vi "Lab Panel V5.20.vi"() -> ()   [LabVIEW 2013] (continued)
                  tunnel: w4670 -> [w4735 _ _]
                  tunnel: w4669 -> [w4733 _ _]
                  tunnel: w4668 -> [w4724 _ _]
                  tunnel: w4667 -> [w4722 _ _]
                  tunnel: w4666 -> [w4716 _ _]
                  tunnel: w4665 -> [w4714 _ _]
                  tunnel: w4664 -> [_ w4760 _]
                  tunnel: w4663 -> [_ w4758 _]
                  tunnel: w4662 -> [_ w4749 _]
                  tunnel: w4661 -> [_ w4747 _]
                  frame #0 {
                    n2509 = Merge Signals(w4742, w4741) -> (→"LAB01 AMPS":dynamicdata)
                    n2510 = Merge Signals(w4739, w4738) -> (→"LAB01 VOLTS":dynamicdata)
                    n2511 = Merge Signals(w4719, w4718) -> (→"LAB03 VOLTS":dynamicdata)
                    n2512 = Merge Signals(w4736, w4735, w4734, w4733) -> (→"LAB01 deg C":dynamicdata)
                    n2513 = Merge Signals(w4732, w4731) -> (→"LAB02 AMPS":dynamicdata)
                    n2514 = Merge Signals(w4725, w4724, w4723, w4722) -> (→"LAB02 deg C":dynamicdata)
                    n2515 = Merge Signals(w4717, w4716, w4715, w4714) -> (→"LAB03 deg C":dynamicdata)
                    n2516 = Merge Signals(w4729, w4728) -> (→"LAB02 VOLTS":dynamicdata)
                    n2517 = Merge Signals(w4721, w4720) -> (→"LAB03 AMPS":dynamicdata)
                  }
                  frame #1 {
                    n2518 = Merge Signals(w4752, w4751) -> (→"LAB05 VOLTS":dynamicdata)
                    n2519 = Merge Signals(w4765, w4764) -> (→"LAB04 AMPS":dynamicdata)
                    n2520 = Merge Signals(w4754, w4753) -> (→"LAB05 AMPS":dynamicdata)
                    n2521 = Merge Signals(w4750, w4749, w4748, w4747) -> (→"LAB05 deg C":dynamicdata)
                    n2522 = Merge Signals(w4761, w4760, w4759, w4758) -> (→"LAB04 deg C":dynamicdata)
                    n2523 = Merge Signals(w4763, w4762) -> (→"LAB04 VOLTS":dynamicdata)
                  }
                  frame #2 {
                    n2524 = local read "LAB05 VOLTS"() -> (w4773:dynamicdata)
                    n2525 = local read "LAB04 VOLTS"() -> (w4774:dynamicdata)
                    n2526 = local read "LAB02 VOLTS"() -> (w4776:dynamicdata)
                    n2527 = local read "LAB03 VOLTS"() -> (w4775:dynamicdata)
                    n2528 = local read "LAB05 AMPS"() -> (w4779:dynamicdata)
                    n2529 = local read "LAB01 VOLTS"() -> (w4777:dynamicdata)
                    n2530 = local read "LAB04 AMPS"() -> (w4780:dynamicdata)
                    n2531 = local read "LAB03 deg C"() -> (w4769:dynamicdata)
                    n2532 = local read "LAB03 AMPS"() -> (w4781:dynamicdata)
                    n2533 = local read "LAB04 deg C"() -> (w4768:dynamicdata)
                    n2534 = local read "LAB05 deg C"() -> (w4767:dynamicdata)
                    n2535 = local read "LAB02 AMPS"() -> (w4782:dynamicdata)
                    n2536 = local read "LAB02 deg C"() -> (w4770:dynamicdata)
                    n2537 = local read "LAB01 deg C"() -> (w4771:dynamicdata)
                    n2538 = local read "LAB01 AMPS"() -> (w4783:dynamicdata)
                    n2539 = Merge Signals(w4771, w4770, w4769, w4768, w4767) -> (w4766:dynamicdata)
                    n2540 = Merge Signals(w4783, w4782, w4781, w4780, w4779) -> (w4778:dynamicdata)
                    n2541 = Merge Signals(w4777, w4776, w4775, w4774, w4773) -> (w4772:dynamicdata)
                    n2542 = global write "Global display 3.vi" "graph volts"(w4772) -> ()
                    n2543 = global write "Global display 3.vi" "graph deg C"(w4766) -> ()
                    n2544 = global write "Global display 3.vi" "graph amps"(w4778) -> ()
                  }
                }
              }
            }
          }
          frame #14 {
            # "check for amps fail"
            # "check for cycle test & temperature rise fail conditions"
            n2545 = local read "jig cycle"() -> (w4807:dbl)
            n2546 = local read "on loops"() -> (w4810:dbl)
            n2547 = local read "jig cycle"() -> (w4812:dbl)
            n2548 = Add(x=w4810, y=3.0) -> (x+y=w4808:dbl)
            n2549 = Equal?(x=w4807, y=w4808) -> (x = y?=w4803:bool)
            n2550 = local read "Fail Loops"() -> (w4784:dbl)
            n2551 = Equal?(x=w4812, y=1.0) -> (x = y?=w4805:bool)
            n2552 = global write "Global 1.vi" "fail count"(w4784) -> ()
            n2553 = stacked-sequence {
              tunnel: w4806 -> [w4815 _ _ _ _ _ _ _ _ _]
              tunnel: w4805 -> [w4816 w4836 w4856 w4876 w4896 w4916 w4936 w4956 w4976 w4996]
              tunnel: w4804 -> [w4813 _ _ _ _ _ _ _ _ _]
              tunnel: w4803 -> [w4814 w4835 w4855 w4875 w4895 w4915 w4935 w4955 w4975 w4995]
              tunnel: w4802 -> [_ w4834 _ _ _ _ _ _ _ _]
              tunnel: w4801 -> [_ w4833 _ _ _ _ _ _ _ _]
              tunnel: w4800 -> [_ _ w4854 _ _ _ _ _ _ _]
              tunnel: w4799 -> [_ _ w4853 _ _ _ _ _ _ _]
              tunnel: w4798 -> [_ _ _ w4874 _ _ _ _ _ _]
              tunnel: w4797 -> [_ _ _ w4873 _ _ _ _ _ _]
              tunnel: w4796 -> [_ _ _ _ w4894 _ _ _ _ _]
              tunnel: w4795 -> [_ _ _ _ w4893 _ _ _ _ _]
              tunnel: w4794 -> [_ _ _ _ _ w4914 _ _ _ _]
              tunnel: w4793 -> [_ _ _ _ _ w4913 _ _ _ _]
              tunnel: w4792 -> [_ _ _ _ _ _ w4934 _ _ _]
              tunnel: w4791 -> [_ _ _ _ _ _ w4933 _ _ _]
              tunnel: w4790 -> [_ _ _ _ _ _ _ w4954 _ _]
              tunnel: w4789 -> [_ _ _ _ _ _ _ w4953 _ _]
              tunnel: w4788 -> [_ _ _ _ _ _ _ _ w4974 _]
              tunnel: w4787 -> [_ _ _ _ _ _ _ _ w4973 _]
              tunnel: w4786 -> [_ _ _ _ _ _ _ _ _ w4994]
              tunnel: w4785 -> [_ _ _ _ _ _ _ _ _ w4993]
              frame #0 {
                # "LAB01-1"
                n2554 = case shown="True" w4813 {
                  tunnel: w4816 -> [_ w4829]
                  tunnel: w4815 -> [_ w4826]
                  tunnel: w4814 -> [_ w4825]
                  frame False {
                  }
                  frame True {
                    n2555 = local read "TEMP START LAB01-1"() -> (w4831:cluster{"TL":dbl, "TN":dbl})
                    n2556 = local read "RESULT LAB01-1"() -> (w4820:bool)
                    n2557 = local read "FAIL LAB01-1"() -> (w4823:cluster{"LO":dbl, "HI":dbl})
                    n2558 = local read "SET LAB01-1"() -> (w4827:T5)
                    n2559 = local read "TDMS LAB01-1"() -> (w4830:refnum<k34>)
                    n2560 = local read "DISP LAB01-1"() -> (w4828:T4)
                    n2561 = local read "SIG LAB01-1"() -> (w4832:T2)
                    n2562 = Bundle("FAIL LAB01-1"=w4823, "SIG LAB01-1"=w4832, "TEMP START LAB01-1"=w4831, "DISP LAB01-1"=w4828, "SET LAB01-1"=w4827, "TDMS LAB01-1"=w4830) -> (w4817:T32)  [unwired: 1 in]
                    n2563 = call "sub vi - cycle&temp fail v7.vi"("Amps Lo?"=w4829, "Input Cluster"=w4817, "SELECT"=w4826, "Amps Hi?"=w4825, "Result In"=w4820) -> ("(FAIL) out"=w4822:cluster{"FAIL LO":dbl, "FAIL HI":dbl}, "(DISP) out"=w4818:T4, "T-RISE"=w4819:cluster{"T-RISE (L)":dbl, "T-RISE (N)":dbl}, "Result Out"=w4821:bool, "file error"=w4824:errorcluster)  [unwired: 10 in]
                    n2564 = local write "TEMP RISE LAB01-1"(w4819) -> ()
                    n2565 = local write "FAIL LAB01-1"(w4822) -> ()
                    n2566 = local write "DISP LAB01-1"(w4818) -> ()
                    n2567 = local write "RESULT LAB01-1"(w4821) -> ()
                    n2568 = local write "data file error"(w4824) -> ()
                  }
                }
              }
              frame #1 {
                # "LAB01-2"
                n2569 = case shown="True" w4834 {
                  tunnel: w4836 -> [_ w4849]
                  tunnel: w4833 -> [_ w4846]
                  tunnel: w4835 -> [_ w4845]
                  frame False {
                  }
                  frame True {
                    n2570 = local read "TEMP START LAB01-2"() -> (w4851:cluster{"TL":dbl, "TN":dbl})
                    n2571 = local read "FAIL LAB01-2"() -> (w4842:cluster{"LO":dbl, "HI":dbl})
                    n2572 = local read "SET LAB01-2"() -> (w4847:T5)
                    n2573 = local read "TDMS LAB01-2"() -> (w4850:refnum<k34>)
                    n2574 = local read "DISP LAB01-2"() -> (w4848:T4)
                    n2575 = local read "RESULT LAB01-2"() -> (w4839:bool)
                    n2576 = local read "SIG LAB01-2"() -> (w4852:T2)
                    n2577 = Bundle("FAIL LAB01-2"=w4842, "SIG LAB01-2"=w4852, "TEMP START LAB01-2"=w4851, "DISP LAB01-2"=w4848, "SET LAB01-2"=w4847, "TDMS LAB01-2"=w4850) -> (w4837:T33)  [unwired: 1 in]
                    n2578 = call "sub vi - cycle&temp fail v7.vi"("Amps Lo?"=w4849, "Input Cluster"=w4837, "SELECT"=w4846, "Amps Hi?"=w4845, "Result In"=w4839) -> ("(FAIL) out"=w4841:cluster{"FAIL LO":dbl, "FAIL HI":dbl}, "(DISP) out"=w4844:T4, "T-RISE"=w4838:cluster{"T-RISE (L)":dbl, "T-RISE (N)":dbl}, "Result Out"=w4840:bool, "file error"=w4843:errorcluster)  [unwired: 10 in]
                    n2579 = local write "TEMP RISE LAB01-2"(w4838) -> ()
                    n2580 = local write "FAIL LAB01-2"(w4841) -> ()
                    n2581 = local write "DISP LAB01-2"(w4844) -> ()
                    n2582 = local write "RESULT LAB01-2"(w4840) -> ()
                    n2583 = local write "data file error"(w4843) -> ()
                  }
                }
              }
              frame #2 {
                # "LAB02-1"
                n2584 = case shown="True" w4854 {
                  tunnel: w4856 -> [_ w4869]
                  tunnel: w4853 -> [_ w4866]
                  tunnel: w4855 -> [_ w4865]
                  frame False {
                  }
                  frame True {
                    n2585 = local read "TEMP START LAB02-1"() -> (w4871:cluster{"TL":dbl, "TN":dbl})
                    n2586 = local read "FAIL LAB02-1"() -> (w4862:cluster{"LO":dbl, "HI":dbl})
                    n2587 = local read "SET LAB02-1"() -> (w4867:T5)
                    n2588 = local read "TDMS LAB02-1"() -> (w4870:refnum<k34>)
                    n2589 = local read "DISP LAB02-1"() -> (w4868:T4)
                    n2590 = local read "SIG LAB02-1"() -> (w4872:T2)
                    n2591 = local read "RESULT LAB02-1"() -> (w4859:bool)
                    n2592 = Bundle("FAIL LAB02-1"=w4862, "SIG LAB02-1"=w4872, "TEMP START LAB02-1"=w4871, "DISP LAB02-1"=w4868, "SET LAB02-1"=w4867, "TDMS LAB02-1"=w4870) -> (w4857:T34)  [unwired: 1 in]
                    n2593 = call "sub vi - cycle&temp fail v7.vi"("Amps Lo?"=w4869, "Input Cluster"=w4857, "SELECT"=w4866, "Amps Hi?"=w4865, "Result In"=w4859) -> ("(FAIL) out"=w4861:cluster{"FAIL LO":dbl, "FAIL HI":dbl}, "(DISP) out"=w4864:T4, "T-RISE"=w4858:cluster{"T-RISE (L)":dbl, "T-RISE (N)":dbl}, "Result Out"=w4860:bool, "file error"=w4863:errorcluster)  [unwired: 10 in]
                    n2594 = local write "TEMP RISE LAB02-1"(w4858) -> ()
                    n2595 = local write "FAIL LAB02-1"(w4861) -> ()
                    n2596 = local write "DISP LAB02-1"(w4864) -> ()
                    n2597 = local write "RESULT LAB02-1"(w4860) -> ()
                    n2598 = local write "data file error"(w4863) -> ()
                  }
                }
              }
              frame #3 {
                # "LAB02-2"
                n2599 = case shown="True" w4874 {
                  tunnel: w4876 -> [_ w4889]
                  tunnel: w4873 -> [_ w4886]
                  tunnel: w4875 -> [_ w4885]
                  frame False {
                  }
                  frame True {
                    n2600 = local read "TEMP START LAB02-2"() -> (w4891:cluster{"TL":dbl, "TN":dbl})
                    n2601 = local read "FAIL LAB02-2"() -> (w4882:cluster{"LO":dbl, "HI":dbl})
                    n2602 = local read "SET LAB02-2"() -> (w4887:T5)
                    n2603 = local read "TDMS LAB02-2"() -> (w4890:refnum<k34>)
                    n2604 = local read "DISP LAB02-2"() -> (w4888:T4)
                    n2605 = local read "SIG LAB02-2"() -> (w4892:T2)
                    n2606 = local read "RESULT LAB02-2"() -> (w4879:bool)
                    n2607 = Bundle("FAIL LAB02-2"=w4882, "SIG LAB02-2"=w4892, "TEMP START LAB02-2"=w4891, "DISP LAB02-2"=w4888, "SET LAB02-2"=w4887, "TDMS LAB02-2"=w4890) -> (w4877:T35)  [unwired: 1 in]
                    n2608 = call "sub vi - cycle&temp fail v7.vi"("Amps Lo?"=w4889, "Input Cluster"=w4877, "SELECT"=w4886, "Amps Hi?"=w4885, "Result In"=w4879) -> ("(FAIL) out"=w4881:cluster{"FAIL LO":dbl, "FAIL HI":dbl}, "(DISP) out"=w4884:T4, "T-RISE"=w4878:cluster{"T-RISE (L)":dbl, "T-RISE (N)":dbl}, "Result Out"=w4880:bool, "file error"=w4883:errorcluster)  [unwired: 10 in]
                    n2609 = local write "TEMP RISE LAB02-2"(w4878) -> ()
                    n2610 = local write "FAIL LAB02-2"(w4881) -> ()
                    n2611 = local write "DISP LAB02-2"(w4884) -> ()
                    n2612 = local write "RESULT LAB02-2"(w4880) -> ()
                    n2613 = local write "data file error"(w4883) -> ()
                  }
                }
              }
              frame #4 {
                # "LAB03-1"
                n2614 = case shown="True" w4894 {
                  tunnel: w4896 -> [_ w4909]
                  tunnel: w4893 -> [_ w4906]
                  tunnel: w4895 -> [_ w4905]
                  frame False {
                  }
                  frame True {
                    n2615 = local read "TEMP START LAB03-1"() -> (w4911:cluster{"TL":dbl, "TN":dbl})
                    n2616 = local read "FAIL LAB03-1"() -> (w4902:cluster{"LO":dbl, "HI":dbl})
                    n2617 = local read "SET LAB03-1"() -> (w4907:T5)
                    n2618 = local read "TDMS LAB03-1"() -> (w4910:refnum<k34>)
                    n2619 = local read "DISP LAB03-1"() -> (w4908:T4)
                    n2620 = local read "SIG LAB03-1"() -> (w4912:T2)
                    n2621 = local read "RESULT LAB03-1"() -> (w4899:bool)
                    n2622 = Bundle("FAIL LAB03-1"=w4902, "SIG LAB03-1"=w4912, "TEMP START LAB03-1"=w4911, "DISP LAB03-1"=w4908, "SET LAB03-1"=w4907, "TDMS LAB03-1"=w4910) -> (w4897:T36)  [unwired: 1 in]
                    n2623 = call "sub vi - cycle&temp fail v7.vi"("Amps Lo?"=w4909, "Input Cluster"=w4897, "SELECT"=w4906, "Amps Hi?"=w4905, "Result In"=w4899) -> ("(FAIL) out"=w4901:cluster{"FAIL LO":dbl, "FAIL HI":dbl}, "(DISP) out"=w4904:T4, "T-RISE"=w4898:cluster{"T-RISE (L)":dbl, "T-RISE (N)":dbl}, "Result Out"=w4900:bool, "file error"=w4903:errorcluster)  [unwired: 10 in]
                    n2624 = local write "TEMP RISE LAB03-1"(w4898) -> ()
                    n2625 = local write "FAIL LAB03-1"(w4901) -> ()
                    n2626 = local write "DISP LAB03-1"(w4904) -> ()
                    n2627 = local write "RESULT LAB03-1"(w4900) -> ()
                    n2628 = local write "data file error"(w4903) -> ()
                  }
                }
              }
              frame #5 {
                # "LAB03-2"
                n2629 = case shown="True" w4914 {
                  tunnel: w4916 -> [_ w4929]
                  tunnel: w4913 -> [_ w4926]
                  tunnel: w4915 -> [_ w4925]
                  frame False {
                  }
                  frame True {
                    n2630 = local read "TEMP START LAB03-2"() -> (w4931:cluster{"TL":dbl, "TN":dbl})
                    n2631 = local read "FAIL LAB03-2"() -> (w4922:cluster{"LO":dbl, "HI":dbl})
                    n2632 = local read "SET LAB03-2"() -> (w4927:T5)
                    n2633 = local read "TDMS LAB03-2"() -> (w4930:refnum<k34>)
                    n2634 = local read "DISP LAB03-2"() -> (w4928:T4)
                    n2635 = local read "RESULT LAB03-2"() -> (w4919:bool)
                    n2636 = local read "SIG LAB03-2"() -> (w4932:T2)
                    n2637 = Bundle("FAIL LAB03-2"=w4922, "SIG LAB03-2"=w4932, "TEMP START LAB03-2"=w4931, "DISP LAB03-2"=w4928, "SET LAB03-2"=w4927, "TDMS LAB03-2"=w4930) -> (w4917:T37)  [unwired: 1 in]
                    n2638 = call "sub vi - cycle&temp fail v7.vi"("Amps Lo?"=w4929, "Input Cluster"=w4917, "SELECT"=w4926, "Amps Hi?"=w4925, "Result In"=w4919) -> ("(FAIL) out"=w4921:cluster{"FAIL LO":dbl, "FAIL HI":dbl}, "(DISP) out"=w4924:T4, "T-RISE"=w4918:cluster{"T-RISE (L)":dbl, "T-RISE (N)":dbl}, "Result Out"=w4920:bool, "file error"=w4923:errorcluster)  [unwired: 10 in]
                    n2639 = local write "FAIL LAB03-2"(w4921) -> ()
                    n2640 = local write "TEMP RISE LAB03-2"(w4918) -> ()
                    n2641 = local write "DISP LAB03-2"(w4924) -> ()
                    n2642 = local write "RESULT LAB03-2"(w4920) -> ()
                    n2643 = local write "data file error"(w4923) -> ()
                  }
                }
              }
              frame #6 {
                # "LAB04-1"
                n2644 = case shown="True" w4934 {
                  tunnel: w4936 -> [_ w4949]
                  tunnel: w4933 -> [_ w4946]
                  tunnel: w4935 -> [_ w4945]
                  frame False {
                  }
                  frame True {
                    n2645 = local read "TEMP START LAB04-1"() -> (w4951:cluster{"TL":dbl, "TN":dbl})
                    n2646 = local read "FAIL LAB04-1"() -> (w4942:cluster{"LO":dbl, "HI":dbl})
                    n2647 = local read "SET LAB04-1"() -> (w4947:T5)
                    n2648 = local read "TDMS LAB04-1"() -> (w4950:refnum<k34>)
                    n2649 = local read "DISP LAB04-1"() -> (w4948:T4)
                    n2650 = local read "SIG LAB04-1"() -> (w4952:T2)
                    n2651 = local read "RESULT LAB04-1"() -> (w4939:bool)
                    n2652 = Bundle("FAIL LAB04-1"=w4942, "SIG LAB04-1"=w4952, "TEMP START LAB04-1"=w4951, "DISP LAB04-1"=w4948, "SET LAB04-1"=w4947, "TDMS LAB04-1"=w4950) -> (w4937:T38)  [unwired: 1 in]
                    n2653 = call "sub vi - cycle&temp fail v7.vi"("Amps Lo?"=w4949, "Input Cluster"=w4937, "SELECT"=w4946, "Amps Hi?"=w4945, "Result In"=w4939) -> ("(FAIL) out"=w4941:cluster{"FAIL LO":dbl, "FAIL HI":dbl}, "(DISP) out"=w4944:T4, "T-RISE"=w4938:cluster{"T-RISE (L)":dbl, "T-RISE (N)":dbl}, "Result Out"=w4940:bool, "file error"=w4943:errorcluster)  [unwired: 10 in]
                    n2654 = local write "FAIL LAB04-1"(w4941) -> ()
                    n2655 = local write "TEMP RISE LAB04-1"(w4938) -> ()
                    n2656 = local write "DISP LAB04-1"(w4944) -> ()
                    n2657 = local write "RESULT LAB04-1"(w4940) -> ()
                    n2658 = local write "data file error"(w4943) -> ()
                  }
                }
              }
              frame #7 {
                # "LAB04-2"
                n2659 = case shown="True" w4954 {
                  tunnel: w4956 -> [_ w4969]
                  tunnel: w4953 -> [_ w4966]
                  tunnel: w4955 -> [_ w4965]
                  frame False {
                  }
                  frame True {
                    n2660 = local read "TEMP START LAB04-2"() -> (w4971:cluster{"TL":dbl, "TN":dbl})
                    n2661 = local read "FAIL LAB04-2"() -> (w4962:cluster{"LO":dbl, "HI":dbl})
                    n2662 = local read "SET LAB04-2"() -> (w4967:T5)
                    n2663 = local read "TDMS LAB04-2"() -> (w4970:refnum<k34>)
                    n2664 = local read "DISP LAB04-2"() -> (w4968:T4)
                    n2665 = local read "SIG LAB04-2"() -> (w4972:T2)
                    n2666 = local read "RESULT LAB04-2"() -> (w4959:bool)
                    n2667 = Bundle("FAIL LAB04-2"=w4962, "SIG LAB04-2"=w4972, "TEMP START LAB04-2"=w4971, "DISP LAB04-2"=w4968, "SET LAB04-2"=w4967, "TDMS LAB04-2"=w4970) -> (w4957:T39)  [unwired: 1 in]
                    n2668 = call "sub vi - cycle&temp fail v7.vi"("Amps Lo?"=w4969, "Input Cluster"=w4957, "SELECT"=w4966, "Amps Hi?"=w4965, "Result In"=w4959) -> ("(FAIL) out"=w4961:cluster{"FAIL LO":dbl, "FAIL HI":dbl}, "(DISP) out"=w4964:T4, "T-RISE"=w4958:cluster{"T-RISE (L)":dbl, "T-RISE (N)":dbl}, "Result Out"=w4960:bool, "file error"=w4963:errorcluster)  [unwired: 10 in]
                    n2669 = local write "TEMP RISE LAB04-2"(w4958) -> ()
                    n2670 = local write "FAIL LAB04-2"(w4961) -> ()
                    n2671 = local write "DISP LAB04-2"(w4964) -> ()
                    n2672 = local write "RESULT LAB04-2"(w4960) -> ()
                    n2673 = local write "data file error"(w4963) -> ()
                  }
                }
              }
              frame #8 {
                # "LAB05-1"
                n2674 = case shown="True" w4974 {
                  tunnel: w4976 -> [_ w4989]
                  tunnel: w4973 -> [_ w4986]
                  tunnel: w4975 -> [_ w4985]
                  frame False {
                  }
                  frame True {
                    n2675 = local read "TEMP START LAB05-1"() -> (w4991:cluster{"TL":dbl, "TN":dbl})
                    n2676 = local read "FAIL LAB05-1"() -> (w4982:cluster{"LO":dbl, "HI":dbl})
                    n2677 = local read "SET LAB05-1"() -> (w4987:T5)
                    n2678 = local read "TDMS LAB05-1"() -> (w4990:refnum<k34>)
                    n2679 = local read "DISP LAB05-1"() -> (w4988:T4)
                    n2680 = local read "SIG LAB05-1"() -> (w4992:T2)
                    n2681 = local read "RESULT LAB05-1"() -> (w4979:bool)
                    n2682 = Bundle("FAIL LAB05-1"=w4982, "SIG LAB05-1"=w4992, "TEMP START LAB05-1"=w4991, "DISP LAB05-1"=w4988, "SET LAB05-1"=w4987, "TDMS LAB05-1"=w4990) -> (w4977:T40)  [unwired: 1 in]
                    n2683 = call "sub vi - cycle&temp fail v7.vi"("Amps Lo?"=w4989, "Input Cluster"=w4977, "SELECT"=w4986, "Amps Hi?"=w4985, "Result In"=w4979) -> ("(FAIL) out"=w4981:cluster{"FAIL LO":dbl, "FAIL HI":dbl}, "(DISP) out"=w4984:T4, "T-RISE"=w4978:cluster{"T-RISE (L)":dbl, "T-RISE (N)":dbl}, "Result Out"=w4980:bool, "file error"=w4983:errorcluster)  [unwired: 10 in]
                    n2684 = local write "TEMP RISE LAB05-1"(w4978) -> ()
                    n2685 = local write "FAIL LAB05-1"(w4981) -> ()
                    n2686 = local write "DISP LAB05-1"(w4984) -> ()
                    n2687 = local write "RESULT LAB05-1"(w4980) -> ()
                    n2688 = local write "data file error"(w4983) -> ()
                  }
                }
              }
              frame #9 {
                # "LAB05-2"
                n2689 = case shown="True" w4994 {
                  tunnel: w4996 -> [_ w5009]
                  tunnel: w4993 -> [_ w5006]
                  tunnel: w4995 -> [_ w5005]
                  frame False {
                  }
                  frame True {
                    n2690 = local read "TEMP START LAB05-2"() -> (w5011:cluster{"TL":dbl, "TN":dbl})
                    n2691 = local read "FAIL LAB05-2"() -> (w5002:cluster{"LO":dbl, "HI":dbl})
                    n2692 = local read "SET LAB05-2"() -> (w5007:T5)
                    n2693 = local read "TDMS LAB05-2"() -> (w5010:refnum<k34>)
                    n2694 = local read "DISP LAB05-2"() -> (w5008:T4)
                    n2695 = local read "SIG LAB05-2"() -> (w5012:T2)
                    n2696 = local read "RESULT LAB05-2"() -> (w4999:bool)
                    n2697 = Bundle("FAIL LAB05-2"=w5002, "SIG LAB05-2"=w5012, "TEMP START LAB05-2"=w5011, "DISP LAB05-2"=w5008, "SET LAB05-2"=w5007, "TDMS LAB05-2"=w5010) -> (w4997:T41)  [unwired: 1 in]
                    n2698 = call "sub vi - cycle&temp fail v7.vi"("Amps Lo?"=w5009, "Input Cluster"=w4997, "SELECT"=w5006, "Amps Hi?"=w5005, "Result In"=w4999) -> ("(FAIL) out"=w5001:cluster{"FAIL LO":dbl, "FAIL HI":dbl}, "(DISP) out"=w5004:T4, "T-RISE"=w4998:cluster{"T-RISE (L)":dbl, "T-RISE (N)":dbl}, "Result Out"=w5000:bool, "file error"=w5003:errorcluster)  [unwired: 10 in]
                    n2699 = local write "TEMP RISE LAB05-2"(w4998) -> ()
                    n2700 = local write "FAIL LAB05-2"(w5001) -> ()
                    n2701 = local write "DISP LAB05-2"(w5004) -> ()
                    n2702 = local write "RESULT LAB05-2"(w5000) -> ()
                    n2703 = local write "data file error"(w5003) -> ()
                  }
                }
              }
            }
          }
          frame #15 {
            # "run calibration routine"
            n2704 = local read "SET (cal)"() -> (w5013:bool)
            n2705 = case shown="True" w5013 {
              frame False {
              }
              frame True {
                n2706 = stacked-sequence {
                  seq-local: [w5014 _ _] -> [_ w5016 _]
                  frame #0 {
                    n2707 = call "CALIBRATION PASSWORD"() -> ("PASSWORD"=w5014:string)  [unwired: 17 in, 2 out]
                  }
                  frame #1 {
                    n2708 = Equal?(x=w5016, y="7777") -> (x = y?=w5015:bool)
                    n2709 = case shown="True" w5015 {
                      frame False {
                      }
                      frame True {
                        n2710 = stacked-sequence {
                          frame #0 {
                            n2711 = local read "Temp Test Cal"() -> (w5018:dbl)
                            n2712 = call "sub vi - calibration v1.vi"("Temp Test Cal"=w5018) -> ()  [unwired: 11 in]
                          }
                          frame #1 {
                            n2713 = call "sub vi - get calibration values v1.vi"() -> ("TEMP REF CAL"=w5019:dbl, "LAB01 (CAL)"=w5024:T14, "LAB02 (CAL)"=w5023:T15, "LAB03 (CAL)"=w5022:T14, "LAB04 (CAL)"=w5021:T14, "calibration file error out"=w5025:errorcluster, "LAB05 (CAL)"=w5020:T14)  [unwired: 9 in]
                            n2714 = local write "TEMP REF cal"(w5019) -> ()
                            n2715 = local write "cal file error out"(w5025) -> ()
                            n2716 = local write "CAL LAB04"(w5021) -> ()
                            n2717 = local write "CAL LAB05"(w5020) -> ()
                            n2718 = local write "CAL LAB01"(w5024) -> ()
                            n2719 = local write "CAL LAB02"(w5023) -> ()
                            n2720 = local write "CAL LAB03"(w5022) -> ()
                          }
                        }
                      }
                    }
                  }
                  frame #2 {
                    n2721 = local write "SET (cal)"(FALSE) -> ()
                  }
                }
              }
            }
          }
          frame #16 {
            # "save certain settings to file"
            n2722 = String To Path(string="c:\\crabtree\\Set Up\\") -> (path=w5028:path)
            n2723 = Build Path(base path=w5028, name or relative path="settings.bin") -> (appended path=w5030:path)
            n2724 = Build Path(base path=w5028, name or relative path="mail.bin") -> (appended path=w5027:path)
            n2725 = Create Folder(path (use dialog)=w5028) -> (error out=w5033:errorcluster)  [unwired: 2 in, 2 out]
            n2726 = call <vilib>:"Clear Errors.vi"("error in (no error)"=w5033) -> ()  [unwired: 6 in, 1 out]
            n2727 = stacked-sequence {
              seq-local: [w5045 _] -> [_ w5058]
              tunnel: w5030 -> [_ w5059]
              tunnel: w5027 -> [_ w5057]
              frame #0 {
                n2728 = local read "C drive data root dir"() -> (w5044:path)
                n2729 = local read "Select COM port"() -> (w5041:refnum<visa-resource-name>)
                n2730 = local read "Network Directory"() -> (w5050:path)
                n2731 = local read "SET LAB05-2"() -> (w5049:T5)
                n2732 = local read "SET LAB05-1"() -> (w5048:T5)
                n2733 = local read "SET LAB04-2"() -> (w5047:T5)
                n2734 = local read "SET LAB03-2"() -> (w5051:T5)
                n2735 = local read "SET LAB04-1"() -> (w5046:T5)
                n2736 = local read "SET LAB03-1"() -> (w5052:T5)
                n2737 = local read "SET LAB02-2"() -> (w5053:T5)
                n2738 = local read "SET LAB02-1"() -> (w5054:T5)
                n2739 = local read "SET LAB01-2"() -> (w5055:T5)
                n2740 = local read "Temp Delay Lps"() -> (w5040:dbl)
                n2741 = local read "Amps Fail level"() -> (w5036:dbl)
                n2742 = local read "Temp Test Cal"() -> (w5037:dbl)
                n2743 = local read "SET LAB01-1"() -> (w5056:T5)
                n2744 = local read "Mail Test File To:"() -> (w5035:string)
                n2745 = local read "Temp Value"() -> (w5039:dbl)
                n2746 = local read "Fail Loops"() -> (w5038:dbl)
                n2747 = local read "Mail Test Fail"() -> (w5034:bool)
                n2748 = local read "RATE (Hz)"() -> (w5043:dbl)
                n2749 = local read "SAMPLES"() -> (w5042:dbl)
                n2750 = Bundle("SET LAB01-1"=w5056, "SET LAB01-2"=w5055, "SET LAB02-1"=w5054, "SET LAB02-2"=w5053, "SET LAB03-1"=w5052, "SET LAB03-2"=w5051, "SET LAB04-1"=w5046, "SET LAB04-2"=w5047, "SET LAB05-1"=w5048, "SET LAB05-2"=w5049, "Network Directory"=w5050, "C drive data root dir"=w5044, "RATE (Hz)"=w5043, "SAMPLES"=w5042, "Select COM port"=w5041, "Temp Delay Lps"=w5040, "Temp Value"=w5039, "Fail Loops"=w5038, "Temp Test Cal"=w5037, "Amps Fail level"=w5036, "Mail Test File To:"=w5035, "Mail Test Fail"=w5034) -> (w5045:T22)  [unwired: 1 in]
              }
              frame #1 {
                n2751 = event shown="[1] \"SET LAB01-1\", \"SET LAB01-2\", \"SET LAB02-1\", \"SET LAB02-2\", \"SET LAB03-1\", \"SET LAB03-2\", \"SET LAB04-1\", \"SET LAB04-2\", \"SET LAB05-1\", \"SET LAB05-2\", \"Network Directory\", \"C drive data root dir\", \"RATE (Hz)\", \"SAMPLES\", \"Select COM port\", \"Temp Delay Lps\", \"Temp Value\", \"Fail Loops\", \"Temp Test Cal\", \"Amps Fail level\", \"Mail Test File To:\", \"Mail Test Fail\": Value Change" {
                  selector: _ -> [_ _ _]
                  dyn-events: _ -> [_ _ _]
                  timeout: 10.0 -> [_ _ _]
                  tunnel: w5059 -> [_ w5061 _]
                  tunnel: w5058 -> [_ w5062 _]
                  tunnel: w5057 -> [_ _ w5073]
                  event Timeout {
                    n2752 = event-data() -> ()  [unwired: 1 in, 3 out]
                  }
                  event "SET LAB01-1", "SET LAB01-2", "SET LAB02-1", "SET LAB02-2", "SET LAB03-1", "SET LAB03-2", "SET LAB04-1", "SET LAB04-2", "SET LAB05-1", "SET LAB05-2", "Network Directory", "C drive data root dir", "RATE (Hz)", "SAMPLES", "Select COM port", "Temp Delay Lps", "Temp Value", "Fail Loops", "Temp Test Cal", "Amps Fail level", "Mail Test File To:", "Mail Test Fail": Value Change {
                    n2753 = event-data() -> ()  [unwired: 1 in, 6 out]
                    n2754 = Open/Create/Replace File(file path (use dialog)=w5061, operation (0:open)=T21."replace or create") -> (refnum out=w5067:refnum<file>, error out=w5066:errorcluster)  [unwired: 4 in, 1 out]
                    n2755 = Write to Binary File(file (use dialog)=w5067, data=w5062, error in=w5066) -> (refnum out=w5065:refnum<file>, error out=w5064:errorcluster)  [unwired: 3 in, 1 out]
                    n2756 = Close File(refnum=w5065, error in=w5064) -> (error out=w5063:errorcluster)  [unwired: 1 out]
                    n2757 = local write "data file error"(w5063) -> ()
                  }
                  event "MAIL SETTINGS.OUT SERVER ADDRESS", "MAIL SETTINGS.FROM ACCOUNT", "MAIL SETTINGS.USER NAME", "MAIL SETTINGS.PASSWORD", "Auto Mail Send", "TO (string):": Value Change {
                    n2758 = event-data() -> ()  [unwired: 1 in, 6 out]
                    n2759 = local read "MAIL SETTINGS"() -> (w5072:T7)
                    n2760 = local read "Auto Mail Send"() -> (w5070:bool)
                    n2761 = local read "TO (string):"() -> (w5069:string)
                    n2762 = Open/Create/Replace File(file path (use dialog)=w5073, operation (0:open)=T21."replace or create") -> (refnum out=w5078:refnum<file>, error out=w5077:errorcluster)  [unwired: 4 in, 1 out]
                    n2763 = Bundle("MAIL SETTINGS"=w5072, "Auto Mail Send"=w5070, "TO (string):"=w5069) -> (w5071:T42)  [unwired: 1 in]
                    n2764 = Write to Binary File(file (use dialog)=w5078, data=w5071, error in=w5077) -> (refnum out=w5076:refnum<file>, error out=w5075:errorcluster)  [unwired: 3 in, 1 out]
                    n2765 = Close File(refnum=w5076, error in=w5075) -> (error out=w5074:errorcluster)  [unwired: 1 out]
                    n2766 = local write "data file error"(w5074) -> ()
                  }
                }
              }
            }
          }
          frame #17 {
            # "mail control"
            n2767 = local read "MAIL SETTINGS"() -> (w5095:T7)
            n2768 = local read "Auto Mail Send"() -> (w5081:bool)
            n2769 = Unbundle(w5095) -> ("OUT SERVER ADDRESS"=w5094:string, "FROM ACCOUNT"=w5093:string, "TEST MAIL"=w5092:bool)  [unwired: 4 out]
            n2770 = stacked-sequence {
              tunnel: "TO (string):" -> [_ w5134]
              tunnel: w5095 -> [w5100 w5133]
              tunnel: w5094 -> [w5099 w5132]
              tunnel: w5093 -> [w5098 w5131]
              tunnel: w5092 -> [w5097 _]
              tunnel: w5081 -> [_ w5130]
              tunnel: w5091 -> [_ w5129]
              tunnel: w5090 -> [_ w5128]
              tunnel: w5089 -> [_ w5127]
              tunnel: w5088 -> [_ w5126]
              tunnel: w5087 -> [_ w5125]
              tunnel: w5086 -> [_ w5124]
              tunnel: w5085 -> [_ w5123]
              tunnel: w5084 -> [_ w5122]
              tunnel: w5083 -> [_ w5121]
              tunnel: w5082 -> [_ w5120]
              tunnel: "TO (string):" -> [w5096 _]
              frame #0 {
                # "mail test"
                n2771 = case shown="True" w5097 {
                  tunnel: w5100 -> [_ w5104]
                  tunnel: w5096 -> [_ w5103]
                  tunnel: w5099 -> [_ w5102]
                  tunnel: w5098 -> [_ w5101]
                  frame False {
                  }
                  frame True {
                    n2772 = stacked-sequence {
                      seq-local: [_ _ w5114 _] -> [_ _ _ w5115]
                      tunnel: w5104 -> [w5107 _ _ w5119]
                      tunnel: w5103 -> [_ _ w5112 _]
                      tunnel: w5102 -> [_ _ w5110 _]
                      tunnel: w5101 -> [_ _ w5111 _]
                      frame #0 {
                        n2773 = Bundle(cluster=w5107, "TEST MAIL STATUS"="TEST START") -> (w5105:T7)  [unwired: 6 in]
                        n2774 = local write "MAIL SETTINGS"(w5105) -> ()
                      }
                      frame #1 {
                        n2775 = Wait (ms)(milliseconds to wait=500) -> ()  [unwired: 1 out]
                      }
                      frame #2 {
                        n2776 = call "sub vi - send mail v5.vi"("TO:"=w5112, "subject"="MAIL TEST FROM LAB PANEL", "from"=w5111, "out going server"=w5110, "message"="TEST MESSAGE") -> ("error out"=w5114:errorcluster)  [unwired: 10 in]
                      }
                      frame #3 {
                        n2777 = Bundle(cluster=w5119, "TEST MAIL"=FALSE, "TEST MAIL STATUS"="TEST END", "mail error"=w5115) -> (w5117:T7)  [unwired: 4 in]
                        n2778 = local write "MAIL SETTINGS"(w5117) -> ()
                      }
                    }
                  }
                }
              }
              frame #1 {
                # "mail report"
                n2779 = stacked-sequence {
                  seq-local: [_ w5177 _ _] -> [_ _ _ w5367]
                  seq-local: [_ _ w5280 _] -> [_ _ _ w5357]
                  seq-local: [w5144 _ _ _] -> [_ w5194 _ _]
                  seq-local: [w5143 _ _ _] -> [_ w5193 _ _]
                  seq-local: [w5141 _ _ _] -> [_ w5191 _ _]
                  seq-local: [w5142 _ _ _] -> [_ w5192 _ _]
                  seq-local: [w5140 _ _ _] -> [_ w5190 _ _]
                  seq-local: [w5139 _ _ _] -> [_ w5185 _ _]
                  seq-local: [w5138 _ _ _] -> [_ w5186 _ _]
                  seq-local: [w5137 _ _ _] -> [_ w5187 _ _]
                  seq-local: [w5136 _ _ _] -> [_ w5188 _ _]
                  seq-local: [w5135 _ _ _] -> [_ w5189 _ _]
                  tunnel: w5134 -> [_ _ _ w5368]
                  tunnel: w5133 -> [_ _ _ w5351]
                  tunnel: w5132 -> [_ _ _ w5365]
                  tunnel: w5131 -> [_ _ _ w5364]
                  tunnel: w5130 -> [w5175 _ _ w5359]
                  tunnel: w5129 -> [_ _ w5310 _]
                  tunnel: w5128 -> [_ _ w5307 _]
                  tunnel: w5127 -> [_ _ w5306 _]
                  tunnel: w5126 -> [_ _ w5305 _]
                  tunnel: w5125 -> [_ _ w5304 _]
                  tunnel: w5124 -> [_ _ w5303 _]
                  tunnel: w5123 -> [_ _ w5302 _]
                  tunnel: w5122 -> [_ _ w5301 _]
                  tunnel: w5121 -> [_ _ w5300 _]
                  tunnel: w5120 -> [_ _ w5299 _]
                  frame #0 {
                    n2780 = case shown="False" w5175 {
                      frame False {
                        n2781 = local write "mail control"("") -> ()
                      }
                      frame True {
                      }
                    }
                    n2782 = local read "SET LAB01-1"() -> (w5174:T5)
                    n2783 = local read "SET LAB01-2"() -> (w5173:T5)
                    n2784 = local read "SET LAB02-1"() -> (w5172:T5)
                    n2785 = local read "SET LAB02-2"() -> (w5171:T5)
                    n2786 = local read "SET LAB03-1"() -> (w5170:T5)
                    n2787 = local read "SET LAB04-1"() -> (w5168:T5)
                    n2788 = local read "SET LAB05-1"() -> (w5166:T5)
                    n2789 = local read "SET LAB03-2"() -> (w5169:T5)
                    n2790 = local read "SET LAB04-2"() -> (w5167:T5)
                    n2791 = local read "SET LAB05-2"() -> (w5165:T5)
                    n2792 = Unbundle(w5170) -> ("DESCRIPTION"=w5150:string)  [unwired: 4 out]
                    n2793 = Unbundle(w5169) -> ("DESCRIPTION"=w5149:string)  [unwired: 4 out]
                    n2794 = Unbundle(w5168) -> ("DESCRIPTION"=w5148:string)  [unwired: 4 out]
                    n2795 = Unbundle(w5165) -> ("DESCRIPTION"=w5145:string)  [unwired: 4 out]
                    n2796 = Unbundle(w5171) -> ("DESCRIPTION"=w5151:string)  [unwired: 4 out]
                    n2797 = Unbundle(w5167) -> ("DESCRIPTION"=w5147:string)  [unwired: 4 out]
                    n2798 = Unbundle(w5174) -> ("DESCRIPTION"=w5163:string)  [unwired: 4 out]
                    n2799 = Unbundle(w5172) -> ("DESCRIPTION"=w5152:string)  [unwired: 4 out]
                    n2800 = Unbundle(w5166) -> ("DESCRIPTION"=w5146:string)  [unwired: 4 out]
                    n2801 = Unbundle(w5173) -> ("DESCRIPTION"=w5153:string)  [unwired: 4 out]
                    n2802 = Concatenate Strings("[LAB05-2/", w5145) -> (w5135:string)
                    n2803 = Concatenate Strings("[LAB05-1/", w5146) -> (w5136:string)
                    n2804 = Concatenate Strings("[LAB04-2/", w5147) -> (w5137:string)
                    n2805 = Concatenate Strings("[LAB03-2/", w5149) -> (w5139:string)
                    n2806 = Concatenate Strings("[LAB04-1/", w5148) -> (w5138:string)
                    n2807 = Concatenate Strings("[LAB03-1/", w5150) -> (w5140:string)
                    n2808 = Concatenate Strings("[LAB01-2/", w5153) -> (w5143:string)
                    n2809 = Concatenate Strings("[LAB02-2/", w5151) -> (w5141:string)
                    n2810 = Concatenate Strings("[LAB01-1/", w5163) -> (w5144:string)
                    n2811 = Concatenate Strings("[LAB02-1/", w5152) -> (w5142:string)
                  }
                  frame #1 {
                    w5198 = "/"
                    w5199 = 2.0
                    n2812 = local read "DISP LAB01-2"() -> (w5278:T4)
                    n2813 = local read "DISP LAB01-1"() -> (w5279:T4)
                    n2814 = local read "DISP LAB02-1"() -> (w5277:T4)
                    n2815 = local read "DISP LAB03-2"() -> (w5274:T4)
                    n2816 = local read "DISP LAB02-2"() -> (w5276:T4)
                    n2817 = local read "DISP LAB03-1"() -> (w5275:T4)
                    n2818 = local read "DISP LAB04-2"() -> (w5272:T4)
                    n2819 = local read "DISP LAB04-1"() -> (w5273:T4)
                    n2820 = local read "DISP LAB05-1"() -> (w5271:T4)
                    n2821 = local read "DISP LAB05-2"() -> (w5270:T4)
                    n2822 = Unbundle(w5278) -> ("CYCLE"=w5262:dbl, "MINS"=w5261:dbl, "STATUS"=w5258:string)
                    n2823 = Unbundle(w5279) -> ("CYCLE"=w5267:dbl, "MINS"=w5266:dbl, "STATUS"=w5263:string)
                    n2824 = Unbundle(w5277) -> ("CYCLE"=w5255:dbl, "MINS"=w5254:dbl, "STATUS"=w5253:string)
                    n2825 = Unbundle(w5274) -> ("CYCLE"=w5242:dbl, "MINS"=w5241:dbl, "STATUS"=w5238:string)
                    n2826 = Unbundle(w5275) -> ("CYCLE"=w5247:dbl, "MINS"=w5246:dbl, "STATUS"=w5243:string)
                    n2827 = Unbundle(w5276) -> ("CYCLE"=w5252:dbl, "MINS"=w5251:dbl, "STATUS"=w5248:string)
                    n2828 = Unbundle(w5273) -> ("CYCLE"=w5237:dbl, "MINS"=w5236:dbl, "STATUS"=w5233:string)
                    n2829 = Unbundle(w5272) -> ("CYCLE"=w5232:dbl, "MINS"=w5231:dbl, "STATUS"=w5228:string)
                    n2830 = Unbundle(w5271) -> ("CYCLE"=w5227:dbl, "MINS"=w5226:dbl, "STATUS"=w5223:string)
                    n2831 = Unbundle(w5270) -> ("CYCLE"=w5269:dbl, "MINS"=w5268:dbl, "STATUS"=w5220:string)
                    n2832 = Number To Decimal String(number=w5255) -> (decimal integer string=w5257:string)  [unwired: 1 in]
                    n2833 = Number To Decimal String(number=w5252) -> (decimal integer string=w5250:string)  [unwired: 1 in]
                    n2834 = Number To Decimal String(number=w5247) -> (decimal integer string=w5245:string)  [unwired: 1 in]
                    n2835 = Number To Decimal String(number=w5262) -> (decimal integer string=w5260:string)  [unwired: 1 in]
                    n2836 = Number To Decimal String(number=w5242) -> (decimal integer string=w5240:string)  [unwired: 1 in]
                    n2837 = Number To Decimal String(number=w5267) -> (decimal integer string=w5265:string)  [unwired: 1 in]
                    n2838 = Number To Decimal String(number=w5269) -> (decimal integer string=w5222:string)  [unwired: 1 in]
                    n2839 = Number To Decimal String(number=w5237) -> (decimal integer string=w5235:string)  [unwired: 1 in]
                    n2840 = Number To Decimal String(number=w5232) -> (decimal integer string=w5230:string)  [unwired: 1 in]
                    n2841 = Number To Decimal String(number=w5227) -> (decimal integer string=w5225:string)  [unwired: 1 in]
                    n2842 = Number To Fractional String(number=w5254, precision (6)=w5199) -> (F-format string=w5256:string)  [unwired: 2 in]
                    n2843 = Number To Fractional String(number=w5241, precision (6)=w5199) -> (F-format string=w5239:string)  [unwired: 2 in]
                    n2844 = Number To Fractional String(number=w5251, precision (6)=w5199) -> (F-format string=w5249:string)  [unwired: 2 in]
                    n2845 = Number To Fractional String(number=w5246, precision (6)=w5199) -> (F-format string=w5244:string)  [unwired: 2 in]
                    n2846 = Number To Fractional String(number=w5231, precision (6)=w5199) -> (F-format string=w5229:string)  [unwired: 2 in]
                    n2847 = Number To Fractional String(number=w5236, precision (6)=w5199) -> (F-format string=w5234:string)  [unwired: 2 in]
                    n2848 = Number To Fractional String(number=w5261, precision (6)=w5199) -> (F-format string=w5259:string)  [unwired: 2 in]
                    n2849 = Number To Fractional String(number=w5226, precision (6)=w5199) -> (F-format string=w5224:string)  [unwired: 2 in]
                    n2850 = Number To Fractional String(number=w5266, precision (6)=w5199) -> (F-format string=w5264:string)  [unwired: 2 in]
                    n2851 = Number To Fractional String(number=w5268, precision (6)=w5199) -> (F-format string=w5221:string)  [unwired: 2 in]
                    n2852 = Concatenate Strings(w5198, w5240, w5198, w5239, w5198, w5238) -> (w5214:string)
                    n2853 = Concatenate Strings(w5198, w5235, w5198, w5234, w5198, w5233) -> (w5213:string)
                    n2854 = Concatenate Strings(w5198, w5230, w5198, w5229, w5198, w5228) -> (w5212:string)
                    n2855 = Concatenate Strings(w5198, w5225, w5198, w5224, w5198, w5223) -> (w5211:string)
                    n2856 = Concatenate Strings(w5198, w5222, w5198, w5221, w5198, w5220) -> (w5210:string)
                    n2857 = Concatenate Strings(w5198, w5265, w5198, w5264, w5198, w5263) -> (w5219:string)
                    n2858 = Concatenate Strings(w5198, w5245, w5198, w5244, w5198, w5243) -> (w5215:string)
                    n2859 = Concatenate Strings(w5198, w5260, w5198, w5259, w5198, w5258) -> (w5218:string)
                    n2860 = Concatenate Strings(w5198, w5257, w5198, w5256, w5198, w5253) -> (w5217:string)
                    n2861 = Concatenate Strings(w5198, w5250, w5198, w5249, w5198, w5248) -> (w5216:string)
                    n2862 = Concatenate Strings("]", "\r") -> (w5195:string)
                    n2863 = Concatenate Strings(w5190, w5215, w5195) -> (w5205:string)
                    n2864 = Concatenate Strings(w5192, w5217, w5195) -> (w5207:string)
                    n2865 = Concatenate Strings(w5191, w5216, w5195) -> (w5206:string)
                    n2866 = Concatenate Strings(w5187, w5212, w5195) -> (w5202:string)
                    n2867 = Concatenate Strings(w5188, w5211, w5195) -> (w5203:string)
                    n2868 = Concatenate Strings(w5186, w5213, w5195) -> (w5201:string)
                    n2869 = Concatenate Strings(w5185, w5214, w5195) -> (w5200:string)
                    n2870 = Concatenate Strings(w5189, w5210, w5195) -> (w5204:string)
                    n2871 = Concatenate Strings(w5193, w5218, w5195) -> (w5208:string)
                    n2872 = Concatenate Strings(w5194, w5219, w5195) -> (w5209:string)
                    n2873 = Concatenate Strings(w5209, w5208, w5207, w5206, w5205, w5200, w5201, w5202, w5203, w5204) -> (w5178:string)
                    n2874 = Concatenate Strings("[PANEL/", "DESC/", "CYCLES/", "MINS/", "STATUS]", "\r", w5178) -> (w5177:string)
                    "MAIL REPORT" <- w5177
                    n2875 = global write "Global display 3.vi" "log all"(w5177) -> ()
                  }
                  frame #2 {
                    w5308 = "END"
                    n2876 = local read "mail control"() -> (w5309:string)
                    n2877 = case shown="False" w5304 {
                      tunnel: w5309 -> [w5333 _]
                      tunnel: w5308 -> [w5332 _]
                      tunnel: [w5331 FALSE] -> w5294
                      frame False {
                        n2878 = Equal?(x=w5333, y=w5332) -> (x = y?=w5331:bool)
                      }
                      frame True {
                      }
                    }
                    n2879 = case shown="False" w5310 {
                      tunnel: w5309 -> [w5349 _]
                      tunnel: w5308 -> [w5348 _]
                      tunnel: [w5347 FALSE] -> w5298
                      frame False {
                        n2880 = Equal?(x=w5349, y=w5348) -> (x = y?=w5347:bool)
                      }
                      frame True {
                      }
                    }
                    n2881 = case shown="False" w5307 {
                      tunnel: w5309 -> [w5345 _]
                      tunnel: w5308 -> [w5344 _]
                      tunnel: [w5343 FALSE] -> w5297
                      frame False {
                        n2882 = Equal?(x=w5345, y=w5344) -> (x = y?=w5343:bool)
                      }
                      frame True {
                      }
                    }
                    n2883 = case shown="False" w5305 {
                      tunnel: w5309 -> [w5337 _]
                      tunnel: w5308 -> [w5336 _]
                      tunnel: [w5335 FALSE] -> w5295
                      frame False {
                        n2884 = Equal?(x=w5337, y=w5336) -> (x = y?=w5335:bool)
                      }
                      frame True {
                      }
                    }
                    n2885 = case shown="False" w5306 {
                      tunnel: w5309 -> [w5341 _]
                      tunnel: w5308 -> [w5340 _]
                      tunnel: [w5339 FALSE] -> w5296
                      frame False {
                        n2886 = Equal?(x=w5341, y=w5340) -> (x = y?=w5339:bool)
                      }
                      frame True {
                      }
                    }
                    n2887 = Or(x=w5296, y=w5295) -> (x .or. y?=w5287:bool)
                    n2888 = Or(x=w5298, y=w5297) -> (x .or. y?=w5288:bool)
                    n2889 = Or(x=w5288, y=w5287) -> (x .or. y?=w5283:bool)
                    n2890 = case shown="False" w5300 {
                      tunnel: w5309 -> [w5317 _]
                      tunnel: w5308 -> [w5316 _]
                      tunnel: [w5315 FALSE] -> w5289
                      frame False {
                        n2891 = Equal?(x=w5317, y=w5316) -> (x = y?=w5315:bool)
                      }
                      frame True {
                      }
                    }
                    n2892 = case shown="False" w5299 {
                      tunnel: w5309 -> [w5313 _]
                      tunnel: w5308 -> [w5312 _]
                      tunnel: [w5311 FALSE] -> w5293
                      frame False {
                        n2893 = Equal?(x=w5313, y=w5312) -> (x = y?=w5311:bool)
                      }
                      frame True {
                      }
                    }
                    n2894 = case shown="False" w5301 {
                      tunnel: w5309 -> [w5321 _]
                      tunnel: w5308 -> [w5320 _]
                      tunnel: [w5319 FALSE] -> w5290
                      frame False {
                        n2895 = Equal?(x=w5321, y=w5320) -> (x = y?=w5319:bool)
                      }
                      frame True {
                      }
                    }
                    n2896 = case shown="False" w5303 {
                      tunnel: w5309 -> [w5329 _]
